vi "save open anything.vi"(0 "Variant":variant, 1 "file path":path, 2 "Action":T1, 3 "error in (not an error)":errorcluster, 4 "prompt":string, 5 "pattern":string, 6 "advisory dialog? (display:T)":bool=TRUE) -> (7 "Variant out":variant, 8 "new file path":path, 9 "canceled":bool, 10 "error out":errorcluster)   [LabVIEW 2015]
uses:
  file action.ctl
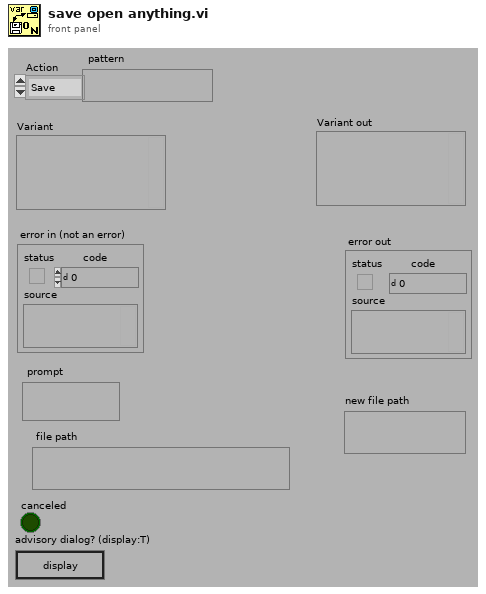
[diagram p1: front panel]
types:
  T1 = typedef "file action.ctl" = enum16{"Save", "Open"}
  T2 = enum16{"open", "open or create", "create or replace", "create", "open (read only)"}
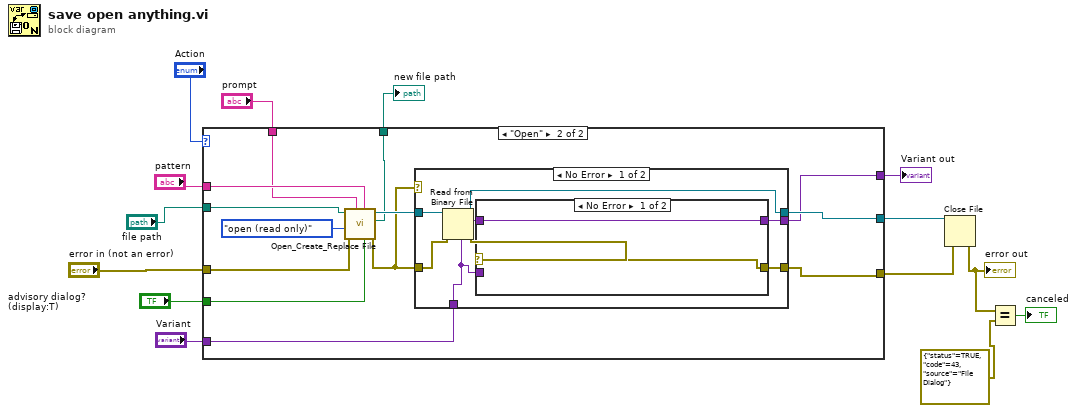
[diagram p0: block diagram]
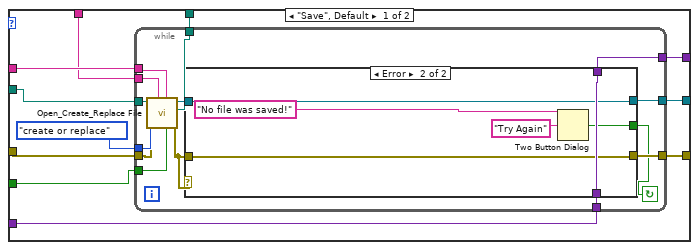
[diagram p2: hidden frame]
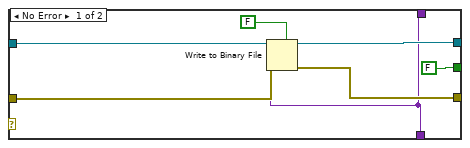
[diagram p3: hidden frame]
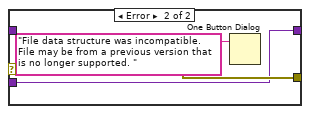
[diagram p4: hidden frame]
diagram:
  n1 = case shown="\"Open\"" "Action" {
    tunnel: [w21 w63] -> w14
    tunnel: [w22 w62] -> w13
    tunnel: "pattern" -> [w24 w64]
    tunnel: "error in (not an error)" -> [w23 w61]
    tunnel: "Variant" -> [w20 w60]
    tunnel: [w18 w59] -> w8
    tunnel: "prompt" -> [w19 w58]
    tunnel: [w17 w55] -> w3
    tunnel: "file path" -> [w16 w54]
    tunnel: "advisory dialog? (display:T)" -> [w15 w53]
    frame "Save", Default {
      n2 = while {
        tunnel: T2."create or replace" ("function (open:0)") -> [w39]
        tunnel: w24 -> [w38]
        tunnel: w23 -> [w37]
        tunnel: [w35] -> w22
        tunnel: [w34] -> w21
        tunnel: w20 -> [w33]
        tunnel: w19 -> [w32]
        tunnel: [w30] -> w18
        tunnel: [w28] -> w17
        tunnel: w16 -> [w27]
        tunnel: w15 -> [w26]
        stop <- w29 continue-if-true
        n3 = call <vilib>:"Open_Create_Replace File.vi"("advisory dialog? (display:T)"=w26, "pattern"=w38, "prompt"=w32, "error in (no error)"=w37, "function (open:0)"=w39, "file path"=w27) -> ("error out"=w31:errorcluster, "new file path"=w28:path, "refnum"=w36:refnum<file>)  [unwired: 2 in, 1 out]
        n4 = case shown="Error" w31 {
          tunnel: w36 -> [w46 w51]
          tunnel: w31 -> [w45 w50]
          tunnel: [w44 w50] -> w35
          tunnel: [w43 w51] -> w34
          tunnel: w33 -> [w42 w52]
          tunnel: [w42 w52] -> w30
          tunnel: [FALSE ("T button?") w47] -> w29
          frame No Error {
            n5 = Write to Binary File(file (use dialog)=w46, data=w42, error in=w45, 5:FALSE ("prepend array or string size? (T)")) -> (refnum out=w43:refnum<file>, error out=w44:errorcluster)  [unwired: 2 in, 1 out]
          }
          frame Error {
            n6 = Two Button Dialog(message="No file was saved!", 2:"Try Again" ("T button name (\"OK\")")) -> (T button?=w47:bool)  [unwired: 1 in]
          }
        }
      }
    }
    frame "Open" {
      n7 = call <vilib>:"Open_Create_Replace File.vi"("advisory dialog? (display:T)"=w53, "pattern"=w64, "prompt"=w58, "error in (no error)"=w61, "function (open:0)"=T2."open (read only)", "file path"=w54) -> ("error out"=w56:errorcluster, "new file path"=w55:path, "refnum"=w57:refnum<file>)  [unwired: 2 in, 1 out]
      n8 = case shown="No Error" w56 {
        tunnel: w57 -> [w73 w80]
        tunnel: w56 -> [w72 w79]
        tunnel: [w71 w80] -> w63
        tunnel: [w69 w79] -> w62
        tunnel: w60 -> [w66 w81]
        tunnel: [w68 w81] -> w59
        frame No Error {
          n9 = Read from Binary File(5:w66, 8:w72, 11:w73) -> (0:w70:errorcluster, 2:w67:variant, 3:w71:refnum<file>)  [unwired: 3 in, 1 out]
          n10 = case shown="No Error" w70 {
            selector: w70 -> [w75 w78]
            tunnel: [w75 w78] -> w69
            tunnel: [w74 w77] -> w68
            tunnel: w67 -> [w74 _]
            tunnel: w66 -> [_ w77]
            frame No Error {
            }
            frame Error {
              n11 = One Button Dialog(message="File data structure was incompatible. File may be from a previous version that is no longer supported. ") -> ()  [unwired: 1 in, 1 out]
            }
          }
        }
        frame Error {
        }
      }
    }
  }
  "Variant out" <- w8
  "new file path" <- w3
  n12 = Close File(refnum=w14, error in=w13) -> (error out=w6:errorcluster)  [unwired: 1 out]
  "error out" <- w6
  n13 = Equal?(x=w6, y=errorcluster {"status"=TRUE, "code"=43, "source"="File Dialog"} ("error out")) -> (x = y?=→"canceled":bool)
